vi "Disconnect.vi"(8 "error in":errorcluster, 11 "WAMP Client in":refnum<class "WAMP Client.lvclass">) -> (0 "error out":errorcluster, 3 "WAMP Client out":refnum<class "WAMP Client.lvclass">)   [LabVIEW 2020, in "wamplv.lvlib" / "WAMP Client.lvclass"]
doc: "This node runs normally even if an error occurred before this node runs."
uses:
  WAMP Client.lvclass
  WAMP Client.lvclass/WAMP Client.ctl
  <vilib>/Utility/error.llb/Error Cluster From Error Code.vi
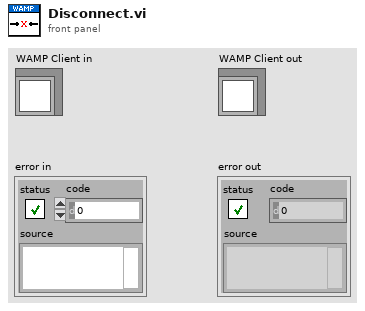
[diagram p1: front panel]
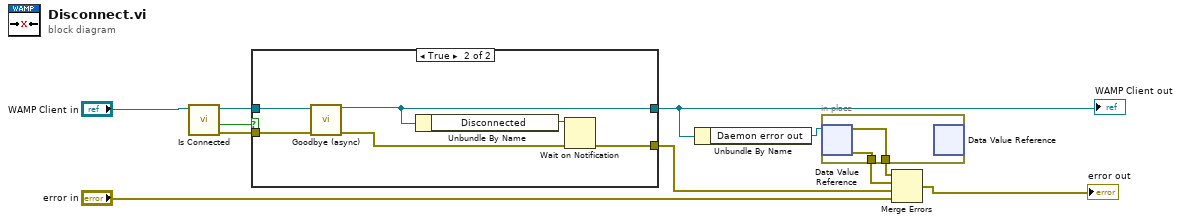
[diagram p0: block diagram]
diagram:
  n1 = call "Is Connected.vi"("WAMP Client in"="WAMP Client in") -> ("error out"=w5:errorcluster, "Is Connected?"=w8:bool, "WAMP Client out"=w6:refnum<class "WAMP Client.lvclass">)  [unwired: 8 in]
  n2 = case shown="True" w8 {
    tunnel: [w13 w17] -> w4
    tunnel: w6 -> [w13 w19]
    tunnel: w5 -> [w12 w18]
    tunnel: [w12 w14] -> w10
    frame False {
    }
    frame True {
      n3 = call-dynamic "Goodbye (async).vi"("error in (no error)"=w18, "WAMP Client in"=w19) -> ("error out"=w15:errorcluster, "WAMP Client out"=w17:refnum<class "WAMP Client.lvclass">)  [unwired: 8 in]
      n4 = Unbundle By Name(w17) -> ("Disconnected"=w16:refnum<notifier>)
      n5 = Wait on Notification(notifier=w16, error in (no error)=w15) -> (error out=w14:errorcluster)  [unwired: 2 in, 3 out]
    }
  }
  "WAMP Client out" <- w4
  n6 = Unbundle By Name(w4) -> ("Daemon error out"=w1:refnum<data-value>)
  n7 = in-place {
    in-place-border: [w21] -> w3
    in-place-border: [w20] -> w2
    n8 = in-place-dvr #1(w1) -> (w20:errorcluster, w21:errorcluster)
    n9 = in-place-dvr #1() -> ()  [unwired: 1 in, 2 out]
  }
  n10 = Merge Errors(w2, w3, w10, "error in") -> (→"error out":errorcluster)
